vi "Handle Remove State Change.vi"(8 "error in (no error)":errorcluster, 10 "State":string, 11 "Routing Channel Ref in":T1 format="%.0x") -> (0 "error out":errorcluster, 2 "State to Display":string, 3 "Routing Channel Ref out":T1 format="%.0x")   [LabVIEW 2020, in "Routing and Faulting System Explorer.lvlib"]
uses:
  Routing and Faulting System Explorer.lvlib
  <vilib>/NI VeriStand/Custom Device API/Custom Device Item Ref.ctl
  Scripting/Routing and Faulting Scripting.lvlib
  <vilib>/NI VeriStand/Custom Device API/Custom Device API.lvlib
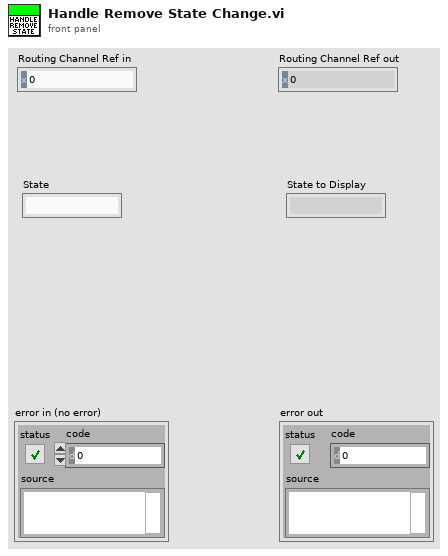
[diagram p1: front panel]
types:
  T1 = typedef "Custom Device API.lvlib/Custom Device Item Ref.ctl" = u64
  T2 = typedef "Routing and Faulting Shared.lvlib/Routing State.ctl" = cluster{"Name":string, "Description":string, "Value":i32, "Connection List":T3[]}
  T3 = typedef "Routing and Faulting Shared.lvlib/Connection.ctl" = cluster{"Module":string, "Source":string, "Destination":string}
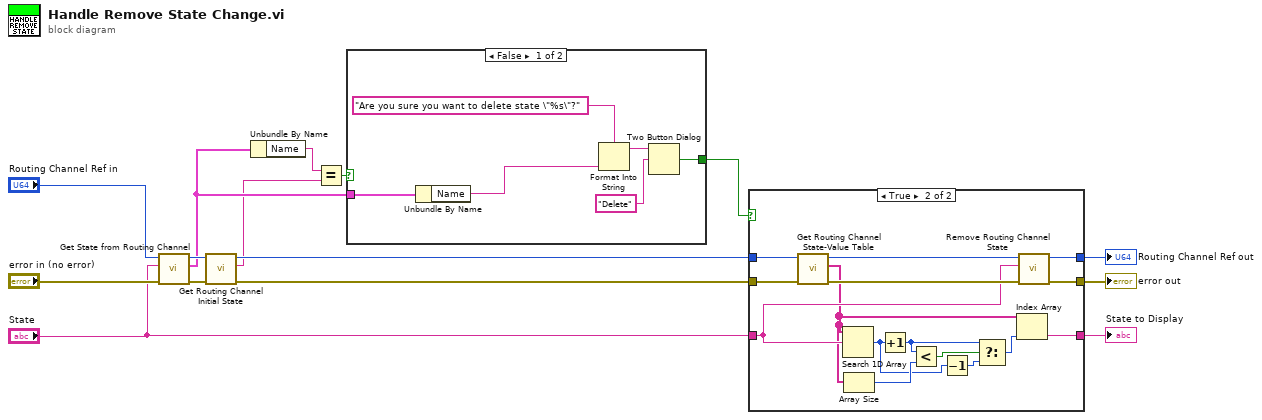
[diagram p0: block diagram]
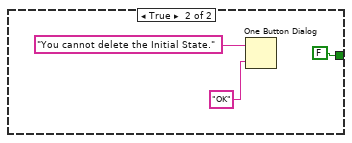
[diagram p2: hidden frame]
diagram:
  n1 = call "Get State from Routing Channel.vi"("error in"="error in (no error)", "state"="State", "routing channel in"="Routing Channel Ref in") -> ("error out"=w12:errorcluster, "state and connections"=w4:T2, "routing channel out"=w6:T1)  [unwired: 6 in]
  n2 = call "Get Routing Channel Initial State.vi"("error in"=w12, "routing channel in"=w6) -> ("error out"=w7:errorcluster, "initial state"=w3:string, "routing channel out"=w5:T1)  [unwired: 7 in]
  n3 = Unbundle By Name(w4) -> ("Name"=w2:string)
  n4 = Equal?(x=w2, y=w3) -> (x = y?=w1:bool)
  n5 = case shown="False" w1 {
    tunnel: w4 -> [w21 _]
    tunnel: [w16 FALSE ("T button?")] -> w10
    frame False {
      n6 = Unbundle By Name(w21) -> ("Name"=w19:string)
      n7 = Format Into String(format string="Are you sure you want to delete state \"%s\"?", w19) -> (resulting string=w18:string)  [unwired: 2 in, 1 out]
      n8 = Two Button Dialog(message=w18, 2:"Delete" ("T button name (\"OK\")")) -> (T button?=w16:bool)  [unwired: 1 in]
    }
    frame True {
      n9 = One Button Dialog(message="You cannot delete the Initial State." ("format string"), button name ("OK")="OK" ("T button name (\"OK\")")) -> ()  [unwired: 1 out]
    }
  }
  n10 = case shown="True" w10 {
    tunnel: w5 -> [w26 w39]
    tunnel: "State" -> [w25 w36]
    tunnel: w7 -> [w27 w40]
    tunnel: [w27 w42] -> w11
    tunnel: [w26 w41] -> w9
    tunnel: [w25 w35] -> w8
    frame False {
    }
    frame True {
      n11 = call "Get Routing Channel State-Value Table.vi"("error in"=w40, "routing channel in"=w39) -> ("error out"=w37:errorcluster, "state names"=w34:string[], "routing channel out"=w38:T1)  [unwired: 6 in, 1 out]
      n12 = Search 1D Array(1D array=w34, element=w36) -> (index of element=w30:i32)  [unwired: 1 in]
      n13 = Array Size(array=w34) -> (size(s)=w33:i32)
      n14 = Increment(x=w30) -> (x+1=w31:i32)
      n15 = Less?(x=w31, y=w33) -> (x < y?=w32:bool)
      n16 = Decrement(x=w30) -> (x-1=w29:i32)
      n17 = Select(t=w31, s=w32, f=w29) -> (s? t:f=w28:i32)
      n18 = Index Array(array=w34, index=w28) -> (element=w35:string)
      n19 = call "Remove Routing Channel State.vi"("error in"=w37, "state"=w36, "routing channel in"=w38) -> ("error out"=w42:errorcluster, "routing channel out"=w41:T1)  [unwired: 7 in]
    }
  }
  "error out" <- w11
  "Routing Channel Ref out" <- w9
  "State to Display" <- w8
